vi "Read Relay.vi"() -> (1 "unsigned 8bit integer":u8, 2 "Boolean array":bool[](array[boolean]))   [LabVIEW 2019, in "Relay-Box.lvclass"]
uses:
  Relay-Box.lvclass
  Relay-Box.lvclass/Relay-Box.ctl
  <instrlib>/FTDI/D2XX/D2XX.lvlib
panel:
  out "error out":errorcluster
  in  "error in (no error)":errorcluster
  out "FT_Status out":u32(ring) items=["FT_OK", "FT_INVALID_HANDLE", "FT_DEVICE_NOT_FOUND", "FT_DEVICE_NOT_OPENED", "FT_IO_ERROR", "FT_INSUFFICIENT_RESOURCES", "FT_INVALID_PARAMETER", "FT_INVALID_BAUD_RATE", "FT_DEVICE_NOT_OPENED_FOR_ERASE", "FT_DEVICE_NOT_OPENED_FOR_WRITE", "FT_FAILED_TO_WRITE_DEVICE", "FT_EEPROM_READ_FAILED", "FT_EEPROM_WRITE_FAILED", "FT_EEPROM_ERASE_FAILED", "FT_EEPROM_NOT_PRESENT", "FT_EEPROM_NOT_PROGRAMMED", "FT_INVALID_ARGS", "FT_NOT_SUPPORTED", "FT_OTHER_ERROR"]
  # "Discharge tip"
  # "0 ohm"
  # "100k ohm"
  # "10M ohm"
  # "1Gohm"
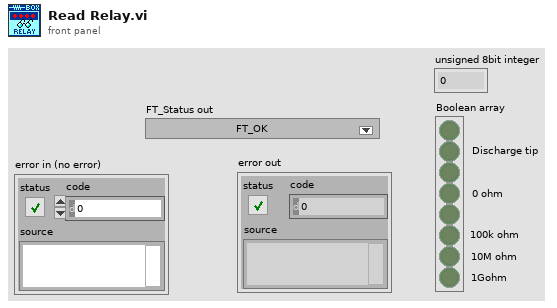
[diagram p1: front panel]
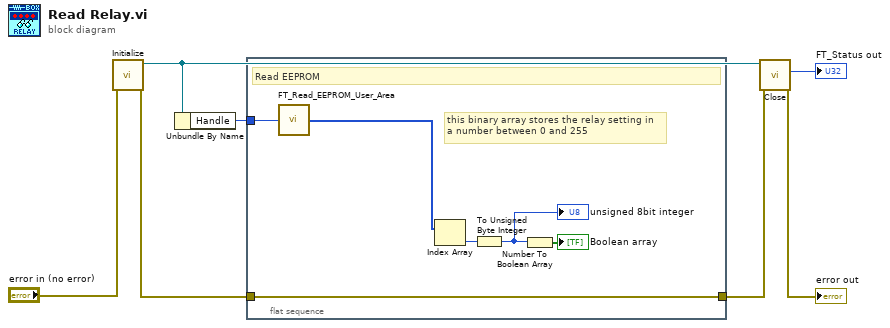
[diagram p0: block diagram]
diagram:
  n1 = call "Initialize.vi"("error in (no error)"="error in (no error)") -> ("error out"=w4:errorcluster, "Relay-Box out"=w6:refnum<class "Relay-Box.lvclass">)  [unwired: 9 in]
  n2 = Unbundle By Name(w6) -> ("Handle"=w7:u32)
  n3 = flat-sequence {
    tunnel: [w11] -> w2
    tunnel: w7 -> [w8]
    tunnel: w4 -> [w11]
    frame #0 {
      # "this binary array stores the relay setting in\na number between 0 and 255"
      # "Read EEPROM"
      n4 = call <instrlib>:"FT_Read_EEPROM_User_Area.vi"("Handle"=w8) -> ("User Area Data"=w9:u8[])  [unwired: 2 out]
      n5 = Index Array(array=w9) -> (element=w10:u8)  [unwired: 1 in]
      n6 = To Unsigned Byte Integer(number=w10) -> (unsigned 8bit integer=w13:u8)
      "unsigned 8bit integer" <- w13
      n7 = Number To Boolean Array(number=w13) -> (Boolean array=→"Boolean array":bool[])
    }
  }
  n8 = call "Close.vi"("error in (no error)"=w2, "Relay-Box in"=w6) -> ("error out"=→"error out":errorcluster, "FT_Status"=→"FT_Status out":u32)  [unwired: 7 in, 1 out]
